vi "solar_misc Rendezvous Wait.vi"(8 "error in (no error)":errorcluster, 9 "Timeout (10000ms)":u32=10000, 11 "Rendezvous in":refnum<queue>) -> (0 "error out":errorcluster, 1 "Timed Out?":bool, 3 "Rendezvous out":refnum<queue>)   [LabVIEW 2018]
doc: "This is a simplified version of NI's rendezvous wait VI."
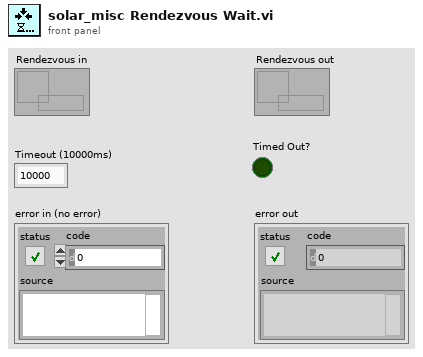
[diagram p1: front panel]
types:
  T1 = cluster{"Size":u32, "Rendezvous":refnum<queue>[]}
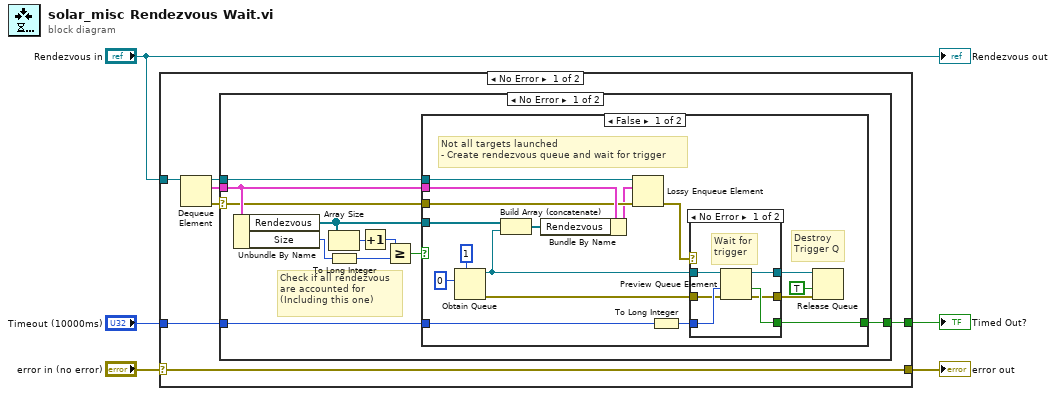
[diagram p0: block diagram]
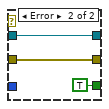
[diagram p2: hidden frame]
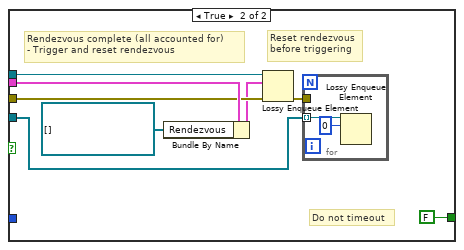
[diagram p3: hidden frame]
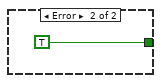
[diagram p4: hidden frame]
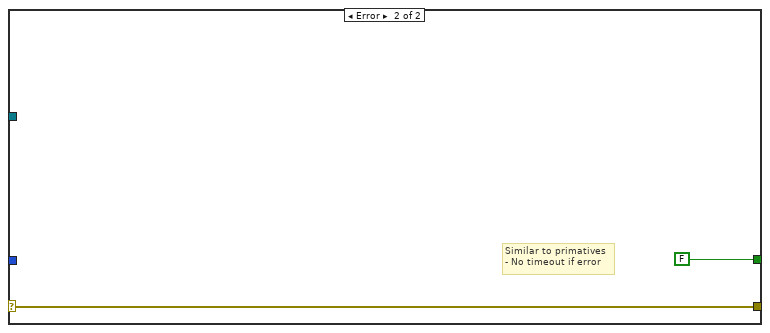
[diagram p5: hidden frame]
diagram:
  n1 = case shown="No Error" "error in (no error)" {
    selector: "error in (no error)" -> [w6 w62]
    tunnel: [w9 FALSE ("timed out?")] -> w5
    tunnel: "Rendezvous in" -> [w8 _]
    tunnel: "Timeout (10000ms)" -> [w7 _]
    tunnel: [w6 w62] -> w3
    frame No Error {
      n2 = Dequeue Element(queue=w8) -> (queue out=w12:refnum<queue>, element=w11:T1, error out=w10:errorcluster)  [unwired: 2 in, 1 out]
      n3 = case shown="No Error" w10 {
        selector: w10 -> [w19 _]
        tunnel: w12 -> [w23 _]
        tunnel: w11 -> [w22 _]
        tunnel: w7 -> [w13 _]
        tunnel: [w18 TRUE ("timed out?")] -> w9
        frame No Error {
          # "Check if all rendezvous\nare accounted for\n(Including this one)"
          n4 = Unbundle By Name(w22) -> ("Rendezvous"=w20:refnum<queue>[], "Size"=w21:u32)
          n5 = Array Size(array=w20) -> (size(s)=w17:i32)
          n6 = To Long Integer(number=w21) -> (32bit integer=w15:i32)
          n7 = Increment(x=w17) -> (x+1=w16:i32)
          n8 = Greater Or Equal?(x=w16, y=w15) -> (x >= y?=w14:bool)
          n9 = case shown="False" w14 {
            tunnel: w23 -> [w40 w55]
            tunnel: w22 -> [w39 w54]
            tunnel: w20 -> [w38 w57]
            tunnel: w19 -> [w37 w53]
            tunnel: [w36 FALSE ("timed out?")] -> w18
            tunnel: w13 -> [w25 _]
            frame False {
              # "Destroy\nTrigger Q"
              # "Not all targets launched\n- Create rendezvous queue and wait for trigger"
              n10 = Obtain Queue(max queue size (-1, unlimited)=1, element data type=u8 0) -> (queue out=w35:refnum<queue>, error out=w34:errorcluster)  [unwired: 3 in, 1 out]
              n11 = Build Array (concatenate)(w38, w35) -> (w29:refnum<queue>[])
              n12 = Bundle By Name(cluster=w39, "Rendezvous"=w29) -> (w30:T1)
              n13 = Lossy Enqueue Element(queue=w40, element=w30, error in (no error)=w37) -> (error out=w26:errorcluster)  [unwired: 3 out]
              n14 = To Long Integer(number=w25) -> (32bit integer=w24:i32)
              n15 = case shown="No Error" w26 {
                tunnel: w24 -> [w46 _]
                tunnel: [w45 TRUE ("timed out?")] -> w36
                tunnel: w35 -> [w44 w49]
                tunnel: w34 -> [w43 w48]
                tunnel: [w42 w49] -> w32
                tunnel: [w41 w48] -> w31
                frame No Error {
                  # "Wait for\ntrigger"
                  n16 = Preview Queue Element(queue=w44, timeout in ms (-1)=w46, error in (no error)=w43) -> (queue out=w42:refnum<queue>, timed out?=w45:bool, error out=w41:errorcluster)  [unwired: 1 out]
                }
                frame Error {
                }
              }
              n17 = Release Queue(queue=w32, force destroy? (F)=TRUE, error in (no error)=w31) -> ()  [unwired: 3 out]
            }
            frame True {
              # "Reset rendezvous\nbefore triggering"
              # "Do not timeout"
              # "Rendezvous complete (all accounted for)\n- Trigger and reset rendezvous"
              n18 = Bundle By Name(cluster=w54, "Rendezvous"=refnum<queue>[] []) -> (w51:T1)
              n19 = Lossy Enqueue Element(queue=w55, element=w51, error in (no error)=w53) -> (error out=w52:errorcluster)  [unwired: 3 out]
              n20 = for {
                tunnel: w57 -> [w59] mode=indexing
                tunnel: w52 -> [_]
                n21 = Lossy Enqueue Element(queue=w59, element=u8 0) -> ()  [unwired: 1 in, 4 out]
              }
            }
          }
        }
        frame Error {
        }
      }
    }
    frame Error {
      # "Similar to primatives\n- No timeout if error"
    }
  }
  "error out" <- w3
  "Timed Out?" <- w5
  "Rendezvous out" <- "Rendezvous in"
